vi "DBL Array to Matlab String.vi"(8 "error in (no error)":errorcluster, 10 "Value":T1, 11 "Variable name":string) -> (0 "error out":errorcluster, 3 "String":string)   [LabVIEW 2012, in "Matlab API.lvlib"]
uses:
  Matlab API.lvlib
  <vilib>/Analysis/Matrix/Datatypes/RealMatrix.ctl
  <vilib>/Analysis/Matrix/NI_Matrix.lvlib
panel:
  out "Array":u8[](array[numeric]) format="%x"
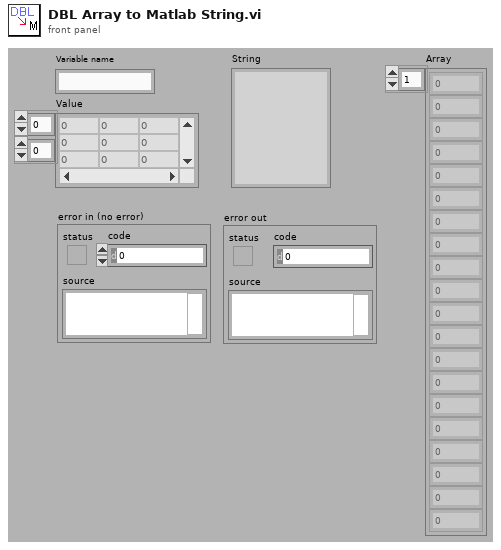
[diagram p1: front panel]
types:
  T1 = typedef "NI_Matrix.lvlib/RealMatrix.ctl" = dbl[][]
  T2 = enum16{"big-endian, network order", "native, host order", "little-endian"}
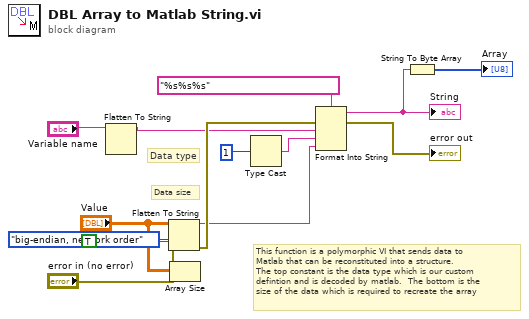
[diagram p0: block diagram]
diagram:
  # "Data size"
  # "Data type"
  # "This function is a polymorphic VI that sends data to\nMatlab that can be reconstituted into a structure.\nThe top constant is the data type which is our custom\ndefintion and is decoded by matlab.  The bottom is the\nsize of the data which is required to recreate the array"
  n1 = Flatten To String(anything="Variable name") -> (data string=w4:string)  [unwired: 1 in, 4 out]
  n2 = Flatten To String(anything="Value", prepend array or string size? (T)=TRUE, byte order (0:big-endian, network order)=T2."big-endian, network order", error in (no error)="error in (no error)") -> (data string=w1:string, error out=w10:errorcluster)  [unwired: 1 out]
  n3 = Array Size(array="Value") -> ()  [unwired: 1 out]
  n4 = Type Cast(x=1 ("input 2")) -> (*(type *) &x=w6:string)  [unwired: 1 out]
  n5 = Format Into String(format string="%s%s%s", error in=w10, w4, w6, w1) -> (resulting string=w7:string, error out=→"error out":errorcluster)  [unwired: 1 in]
  "String" <- w7
  n6 = String To Byte Array(string=w7) -> (unsigned byte array=→"Array":u8[])
